vi "DecryptTileCode_OBSOLETE.vi"(8 "error in (no error)":errorcluster, 11 "TileCode":string) -> (0 "error out":errorcluster, 1 "TileNumber":u8, 2 "found?":bool, 3 "TileCode":u16)   [LabVIEW 2019, in "RT_Game.lvlib" / "Game.lvclass"]
uses:
  Game.lvclass
  <vilib>/Utility/error.llb/Error Cluster From Error Code.vi
  <vilib>/ErrorRing/Error Ring.xnode
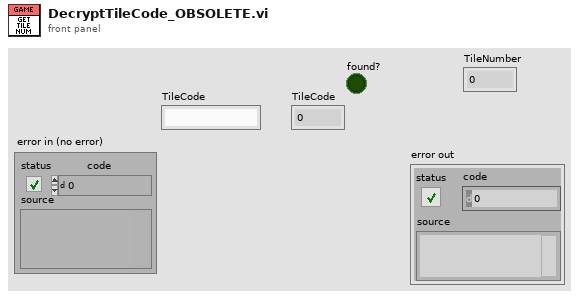
[diagram p1: front panel]
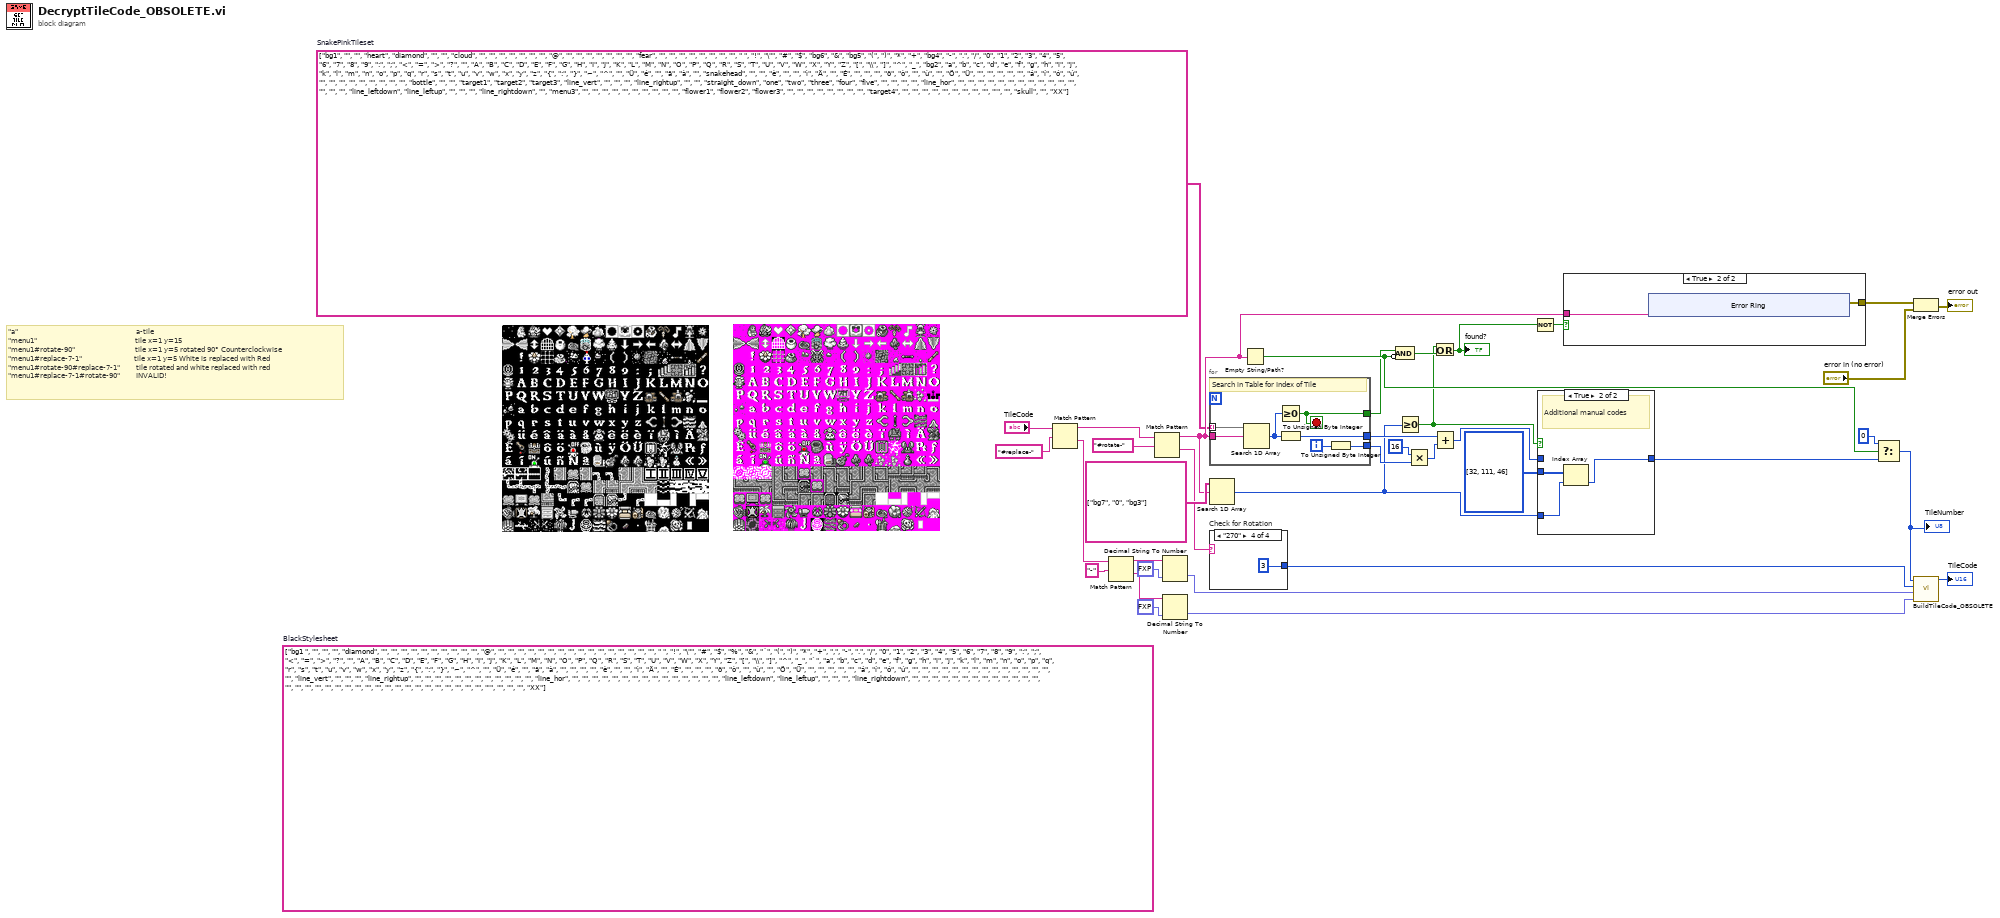
[diagram p0: block diagram]
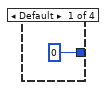
[diagram p2: hidden frame]
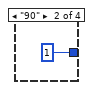
[diagram p3: hidden frame]
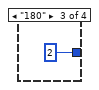
[diagram p4: hidden frame]
diagram:
  (unwired) string[][] [["bg1 ", "", "", "", "diamond", "", "", "", "", "", "", "", "", "", "", "@"], ["", "", "", "", "", "", "", "", "", "", "", "", "", "", "", ""], [" ", "!", "\"", "#", "$", "%", "&", "´", "(", ")", "*", "+", ",", "-", ".", "/"], ["0", "1", "2", "3", "4", "5", "6", "7", "8", "9", ":", ";", "<", "=", ">", "?"], ["", "A", "B", "C", "D", "E", "F", "G", "H", "I", "J", "K", "L", "M", "N", "O"], ["P", "Q", "R", "S", "T", "U", "V", "W", "X", "Y", "Z", "[", "\\", "]", "^", "_"], ["`", "a", "b", "c", "d", "e", "f", "g", "h", "i", "j", "k", "l", "m", "n", "o"], ["p", "q", "r", "s", "t", "u", "v", "w", "x", "y", "z", "{", ":", "}", "~", "^"], ["", "Ü", "é", "", "ä", "à", "", "", "", "", "è", "", "", "ì", "Ä", ""], ["É", "", "", "", "ö", "ò", "", "ù", "", "Ö", "Ü", "", "", "", "", ""], ["á", "í", "ó", "ú", "", "", "", "", "", "", "", "", "", "", "", ""], ["", "", "", "line_vert", "", "", "", "line_rightup", "", "", "", "", "", "", "", ""], ["", "", "", "", "line_hor", "", "", "", "", "", "", "", "", "", "", ""], ["", "", "", "", "line_leftdown", "line_leftup", "", "", "", "line_rightdown", "", "", "", "", "", ""], ["", "", "", "", "", "", "", "", "", "", "", "", "", "", "", ""], ["", "", "", "", "", "", "", "", "", "", "", "'", "", "", "", "XX"]]  # BlackStylesheet
  w1 = string[][] [["bg1", "", "", "heart", "diamond", "", "", "cloud", "", "", "", "", "", "", "", "@"], ["", "", "", "", "", "", "", "fear", "", "", "", "", "", "", "", ""], [" ", "!", "\"", "#", "$", "bg6", "&", "bg5", "(", ")", "*", "+", "bg4", "-", ".", "/"], ["0", "1", "2", "3", "4", "5", "6", "7", "8", "9", ":", ";", "<", "=", ">", "?"], ["", "A", "B", "C", "D", "E", "F", "G", "H", "I", "J", "K", "L", "M", "N", "O"], ["P", "Q", "R", "S", "T", "U", "V", "W", "X", "Y", "Z", "[", "\\", "]", "^", "_"], ["bg2", "a", "b", "c", "d", "e", "f", "g", "h", "i", "j", "k", "l", "m", "n", "o"], ["p", "q", "r", "s", "t", "u", "v", "w", "x", "y", "z", "{", ":", "}", "~", "^"], ["", "Ü", "é", "", "ä", "à", "", "snakehead", "", "", "è", "", "", "ì", "Ä", ""], ["É", "", "", "", "ö", "ò", "", "ù", "", "Ö", "Ü", "", "", "", "", ""], ["á", "í", "ó", "ú", "", "", "", "", "", "", "", "", "", "bottle", "", ""], ["target1", "target2", "target3", "line_vert", "", "", "", "line_rightup", "", "", "straight_down", "one", "two", "three", "four", "five"], ["", "", "", "", "line_hor", "", "", "", "", "", "", "", "", "", "", ""], ["", "", "", "", "line_leftdown", "line_leftup", "", "", "", "line_rightdown", "", "menu3", "", "", "", ""], ["", "", "", "", "", "", "flower1", "flower2", "flower3", "", "", "", "", "", "", ""], ["", "target4", "", "", "", "", "", "", "", "", "", "'", "", "skull", "", "XX"]]  # SnakePinkTileset
  # "\"a\"                                                           a-tile\n\"menu1\"                                                 tile x=1 y=15\n\"menu1#rotate-90\"                              tile x=1 y=5 rotated 90° Counterclockwise\n\"menu1#replace-7-1\"                          tile x=1 y=5 White is replaced with Red\n\"menu1#rotate-90#replace-7-1\"        tile rotated and white replaced with red\n\"menu1#replace-7-1#rotate-90\"        INVALID!"
  n1 = Match Pattern(string="TileCode", regular expression="#replace-" ("search string/char (-)")) -> (before substring=w11:string, after substring=w9:string)  [unwired: 1 in, 2 out]
  n2 = Match Pattern(string=w9, regular expression="-") -> (before substring=w8:string, after substring=w5:string)  [unwired: 1 in, 2 out]
  n3 = Match Pattern(string=w11, regular expression="#rotate-" ("search string/char (-)")) -> (before substring=w17:string, after substring=w16:string)  [unwired: 1 in, 2 out]
  n4 = Decimal String To Number(string=w8, default (0L)=fxp<+,3,3> 0.0) -> (number=w4:fxp<+,3,3>)  [unwired: 1 in, 1 out]
  n5 = Decimal String To Number(string=w5, default (0L)=fxp<+,3,3> 0.0) -> (number=w2:fxp<+,3,3>)  [unwired: 1 in, 1 out]
  n6 = for {
    tunnel: w1 -> [w44] mode=indexing
    tunnel: w17 -> [w43]
    tunnel: [w38] -> w33
    tunnel: [w39] -> w30
    tunnel: [w40] -> w34
    i -> [w42]
    stop <- w40 stop-if-true
    # "Search in Table for Index of Tile"
    n7 = Search 1D Array(1D array=w44, element=w43) -> (index of element=w41:i32)  [unwired: 1 in]
    n8 = Greater Or Equal To 0?(x=w41) -> (x >= 0?=w40:bool)
    n9 = To Unsigned Byte Integer(number=w41) -> (unsigned 8bit integer=w38:u8)
    n10 = To Unsigned Byte Integer(number=w42) -> (unsigned 8bit integer=w39:u8)
  }
  n11 = Search 1D Array(1D array=string[] ["bg7", "0", "bg3"], element=w17) -> (index of element=w23:i32)  [unwired: 1 in]
  n12 = case "Check for Rotation" shown="\"270\"" w16 {
    tunnel: [u8 0 u8 1 u8 2 u8 3] -> w3
    frame Default {
    }
    frame "90" {
    }
    frame "180" {
    }
    frame "270" {
    }
  }
  n13 = Empty String/Path?(string/path=w17) -> (empty?=w37:bool)
  n14 = Compound Arithmetic op=AND(w34, invert w37) -> (w27:bool)
  n15 = Greater Or Equal To 0?(x=w23) -> (x >= 0?=w20:bool)
  n16 = Multiply(x=u8 16, y=w30) -> (x*y=w32:u8)
  n17 = Or(x=w20, y=w27) -> (x .or. y?=w21:bool)
  "found?" <- w21
  n18 = Add(x=w33, y=w32) -> (x+y=w14:u8)
  n19 = Not(x=w21) -> (.not. x?=w25:bool)
  n20 = case shown="True" w20 {
    tunnel: w23 -> [_ w52]
    tunnel: [w49 w51] -> w22
    tunnel: w14 -> [w49 _]
    tunnel: u8[] [32, 111, 46] ("x+y") -> [_ w50]
    frame False {
    }
    frame True {
      # "Additional manual codes"
      n21 = Index Array(array=w50, index=w52) -> (element=w51:u8)
    }
  }
  n22 = case shown="True" w25 {
    tunnel: w17 -> [_ w54]
    tunnel: [_ w53] -> w26
    frame False {
    }
    frame True {
      n23 = xnode "Error Ring"("parameter 0"=w54) -> ("error out"=w53:errorcluster)
    }
  }
  n24 = Select(t=u8 0, s=w37, f=w22) -> (s? t:f=w35:u8)
  "TileNumber" <- w35
  n25 = Merge Errors(w26, "error in (no error)") -> (→"error out":errorcluster)
  n26 = call "BuildTileCode_OBSOLETE.vi"("replace_color"=w2, "color_to_replace"=w4, "rotation"=w3, "tilenumber"=w35) -> ("TileCode"=→"TileCode":u16)  [unwired: 7 in]
